vi "Read Binary Config.vi"(4 "Class Name is Included":bool, 6 "byte order (0:big-endian, network order)":T1(ring), 8 "error in (no error)":errorcluster, 10 "Binary":string, 11 "Const_WFM in":refnum<class "Const_WFM_1D.lvclass">) -> (0 "error out":errorcluster, 2 "Remaining":string, 3 "Const_WFM out":refnum<class "Const_WFM_1D.lvclass">)   [LabVIEW 2021, in "Const_WFM_1D.lvclass"]
uses:
  Const_WFM_1D.lvclass
  Const_WFM_1D.lvclass/Const_WFM_1D.ctl
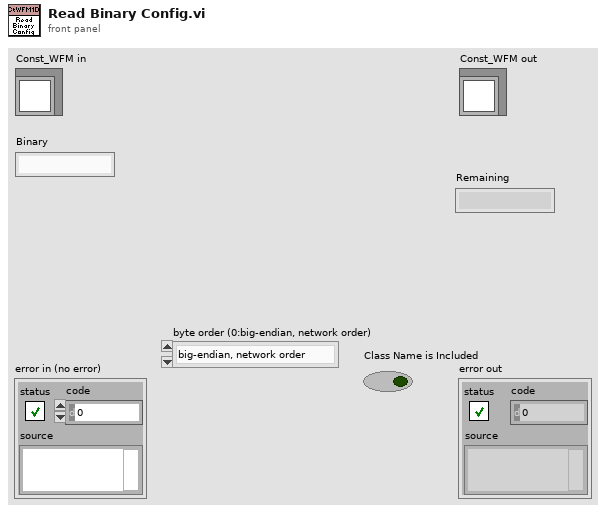
[diagram p1: front panel]
types:
  T1 = enum16{"big-endian, network order", "native, host order", "little-endian"}
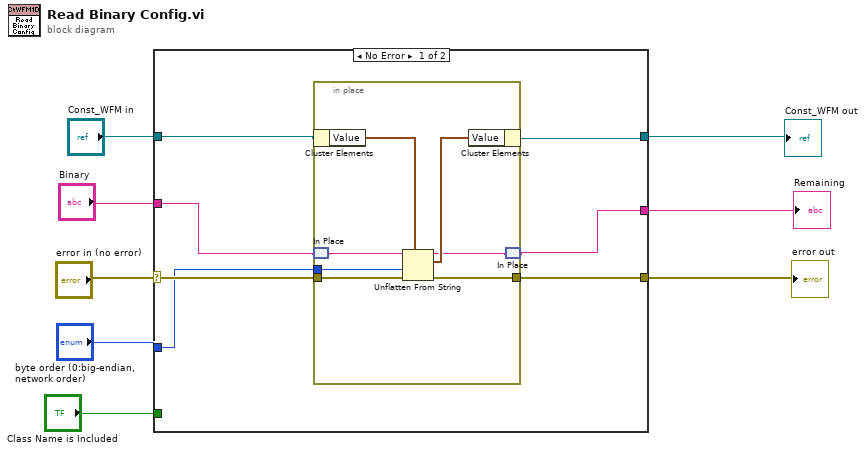
[diagram p0: block diagram]
diagram:
  n1 = case shown="No Error" "error in (no error)" {
    selector: "error in (no error)" -> [w15 w24]
    tunnel: [w14 w24] -> w5
    tunnel: [w11 w25] -> w7
    tunnel: "byte order (0:big-endian, network order)" -> [w13 _]
    tunnel: "Const_WFM in" -> [w12 w25]
    tunnel: "Binary" -> [w10 w23]
    tunnel: [w9 w23] -> w2
    tunnel: "Class Name is Included" -> [_ _]
    frame No Error {
      n2 = in-place {
        in-place-border: w15 -> [w22]
        in-place-border: [w21] -> w14
        in-place-border: w13 -> [w20]
        n3 = in-place-cluster #1(w12) -> ("Value"=w19:waveform(dbl)[])
        n4 = in-place-match #2(w10) -> (w17:string)
        n5 = Unflatten From String(type=w19, binary string=w17, byte order (0:big-endian, network order)=w20, error in (no error)=w22) -> (rest of the binary string=w16:string, value=w18:waveform(dbl)[], error out=w21:errorcluster)  [unwired: 1 in]
        n6 = in-place-cluster #1("Value"=w18) -> (w11:refnum<class "Const_WFM_1D.lvclass">)
        n7 = in-place-match #2(w16) -> (w9:string)
      }
    }
    frame Error {
    }
  }
  "error out" <- w5
  "Const_WFM out" <- w7
  "Remaining" <- w2
